vi "Build Driver Settings Mappings.vi"(8 "error in (no error)":errorcluster, 11 "ArduinoMega2560 in":refnum<class "ArduinoMega2560.lvclass">) -> (0 "error out":errorcluster, 2 "Array":T1[](array[typedef]), 3 "ArduinoMega2560 out":refnum<class "ArduinoMega2560.lvclass">)   [LabVIEW 2023, in "HAF.lvlib" / "ArduinoMega2560.lvclass"]
uses:
  ArduinoMega2560.lvclass
  ArduinoMega2560.lvclass/ArduinoMega2560.ctl
  Setting Map Structure.ctl
  HAF.lvlib
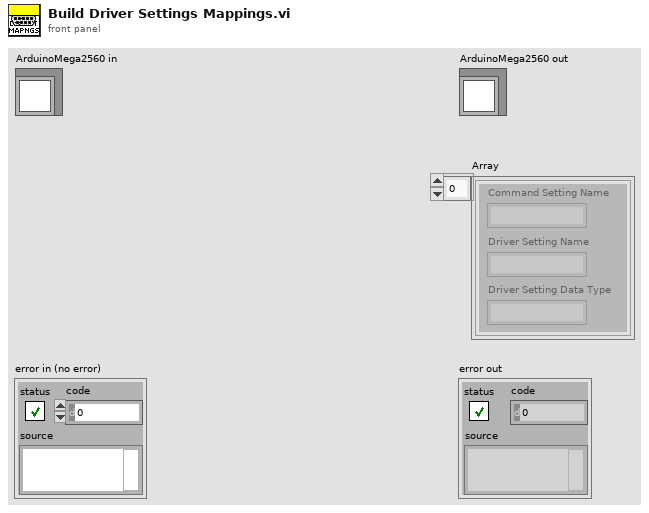
[diagram p1: front panel]
types:
  T1 = typedef "HAF.lvlib/Setting Map Structure.ctl" = cluster{"Command Setting Name":string, "Driver Setting Name":string, "Driver Setting Data Type":string}
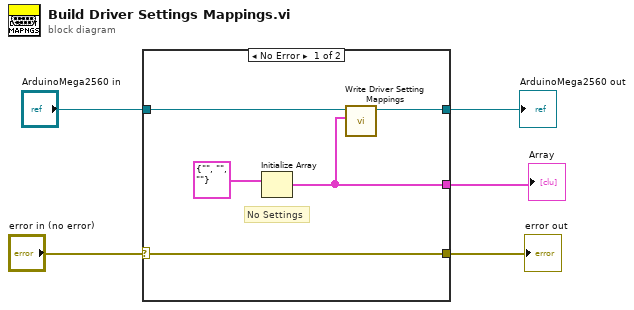
[diagram p0: block diagram]
diagram:
  n1 = case shown="No Error" "error in (no error)" {
    selector: "error in (no error)" -> [w6 w11]
    tunnel: [w8 _] -> w2
    tunnel: "ArduinoMega2560 in" -> [w9 w12]
    tunnel: [w7 w12] -> w3
    tunnel: [w6 w11] -> w1
    frame No Error {
      # "No Settings"
      n2 = Initialize Array(T1 {"Command Setting Name"="", "Driver Setting Name"="", "Driver Setting Data Type"=""} ("Mapping")) -> (w8:T1[])  [unwired: 1 in]
      n3 = call-dynamic "Write Driver Setting Mappings.vi"("Driver Setting Mappings"=w8, "Driver in"=w9) -> ("Driver out"=w7:refnum<class "ArduinoMega2560.lvclass">)  [unwired: 8 in, 1 out]
    }
    frame Error {
    }
  }
  "error out" <- w1
  "ArduinoMega2560 out" <- w3
  "Array" <- w2
